vi "hmi_simRK4serial_variador_2port.vi"() -> ()   [LabVIEW 2017]
uses:
  Control 6.ctl
  <vilib>/Utility/miscctls.llb/LVBoundsTypeDef.ctl
  <vilib>/Instr/_visa.llb/VISA Configure Serial Port (Instr).vi
  <vilib>/MakerHub/LINX/LMH-LINX.lvlib
panel:
  in  "Iniciar fuga":bool
  out "ftselec2":dbl
  out "ftselec1":dbl
  out "Q2":dbl
  out "Q1":dbl
  in  "Simulacion":bool caption="Monitoreo"
  in  "Velocidad":i32(slide) scale=0.0..8333.0
  out "Tiempo":dbl caption="seg" format="%.1f"
  out "Periodo":dbl format="%#_3g"
  in  "FUGA 1":bool
  in  "FUGA 2":bool
  in  "Encendido":bool
  in  "stop":bool
  in  "GUARDAR DATOS EN EXCEL":bool
  in  "Puerto BOMBA":refnum<visa-resource-name>="COM3"
  in  "Puerto sensores":refnum<visa-resource-name>="COM3"
  out "time array":dbl[](array[numeric])
  in  "Tab Control":T1(tab)
  out "Presion de entrada":dbl caption="PSI"
  out "Boolean 2":bool
  out "Boolean":bool
  out "FT1":bool(c317)
  out "valvula 1":bool
  out "valvula 2":bool
  out "TEE 02":bool
  out "TUBERIA 1IN TRAMO 02":bool(c317)
  out "TEE1":bool
  out "Multi-Segment Pipe 2":T2
  out "Multi-Segment Pipe 3":bool(c317)
  out "Multi-Segment Pipe 4":bool(c317)
  out "FT2":bool(c317)
  out "FT 1":dbl caption="L/min"
  out "67.5°":bool
  out "FT 2":dbl caption="L/min"
  out "67.5° 3":bool
  out "45° 3":bool
  out "22.5° 3":bool
  out "90° 3":bool
  out "SENSOR FLUJO 3":bool
  out "45°":bool
  out "22.5°":bool
  out "90°":bool
  out "TANQUE\n FLUIDO:AGUA":dbl(slide) scale=0.0..100.0
  out "SENSOR FLUJO":bool
  out "BOMBA 1/2 HP":bool
  out "codo90":bool
  out "Presion de salida":dbl caption="PSI"
  out "Freq2":dbl
  out "Freq1":dbl
  out "Cluster":T3
  in  "Tab Control 3":enum32{"CAUDAL", "PRESION"}(tab)
  out "Flujo de entrada y salida":cluster{dbl[], dbl[]}[](graph) caption="TRANSMISORES DE FLUJO"
  out "Presion entrada y salida":cluster{dbl[], dbl[]}(graph) caption="TRANSMISORES DE PRESION (PSI)"
  out "Entrada":dbl
  out "Salida":dbl
  in  "Rango de grafica en X":i16(slide)=100 caption="seg" scale=0.0..200.0
  in  "Tab Control 2":T4(tab)
  out "SIMULACION DE Q1 y Q2":cluster{dbl[], dbl[]}[](graph)
  out "SIMULACION DE H2":cluster{"time array":dbl[], dbl[]}(graph)
  in  "Flujo de entrada":dbl=28.44 format="%#_13g"
  in  "Flujo de salida":dbl=26.1 format="%#_13g"
  in  "Rango de grafica":i16(slide)=100 scale=0.0..100.0
  # "INTERFAZ GRAFICA PARA EL MONITOREO DE UN TUBERÍA HIDRÁULICA"
  # "Configuración de comunicación"
  # "Control de Bomba"
  # "Alarmas de detección"
  # "PVC  1\" FLUJO: AGUA"
  # "PVC  1/2\" FLUJO: AGUA"
  # "FUGA 1"
  # "PVC  1/2\" FLUJO: AGUA"
  # "FUGA 2"
  # "PVC  1\" FLUJO: AGUA"
  # "2.5 m"
  # "6 m"
  # "Sensores de Flujo"
  # "Condiciones iniciales"
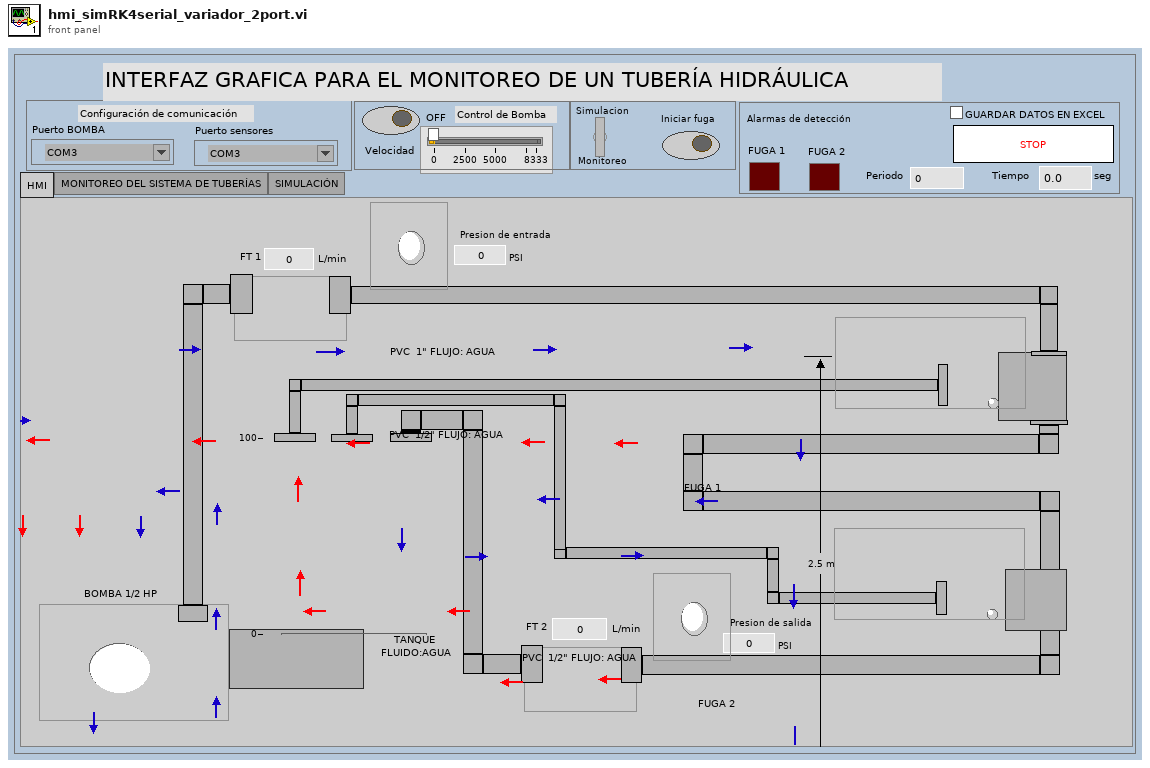
[diagram p1: front panel]
types:
  T1 = enum32{"HMI", "MONITOREO DEL SISTEMA DE TUBERÍAS", "SIMULACIÓN"}
  T2 = typedef "Control 6.ctl" = bool
  T3 = cluster{"FLUJO DE ENTRADA":dbl, "FLUJO DE SALIDA":dbl, "VOLUMEN 1 (L) ":dbl, "VOLUMEN 2 (L) ":dbl}
  T4 = enum32{"FLUJO DE ENTRADA Y SALIDA", "PRESION DE SALIDA"}
  T5 = typedef "LVBoundsTypeDef.ctl" = cluster{"Width":u32, "Height":u32}
  T6 = cluster{"index":i32, "index 2":i32, "index 3":i32, "index 4":i32, "index 5":i32, "index 6":i32, i32, i32}
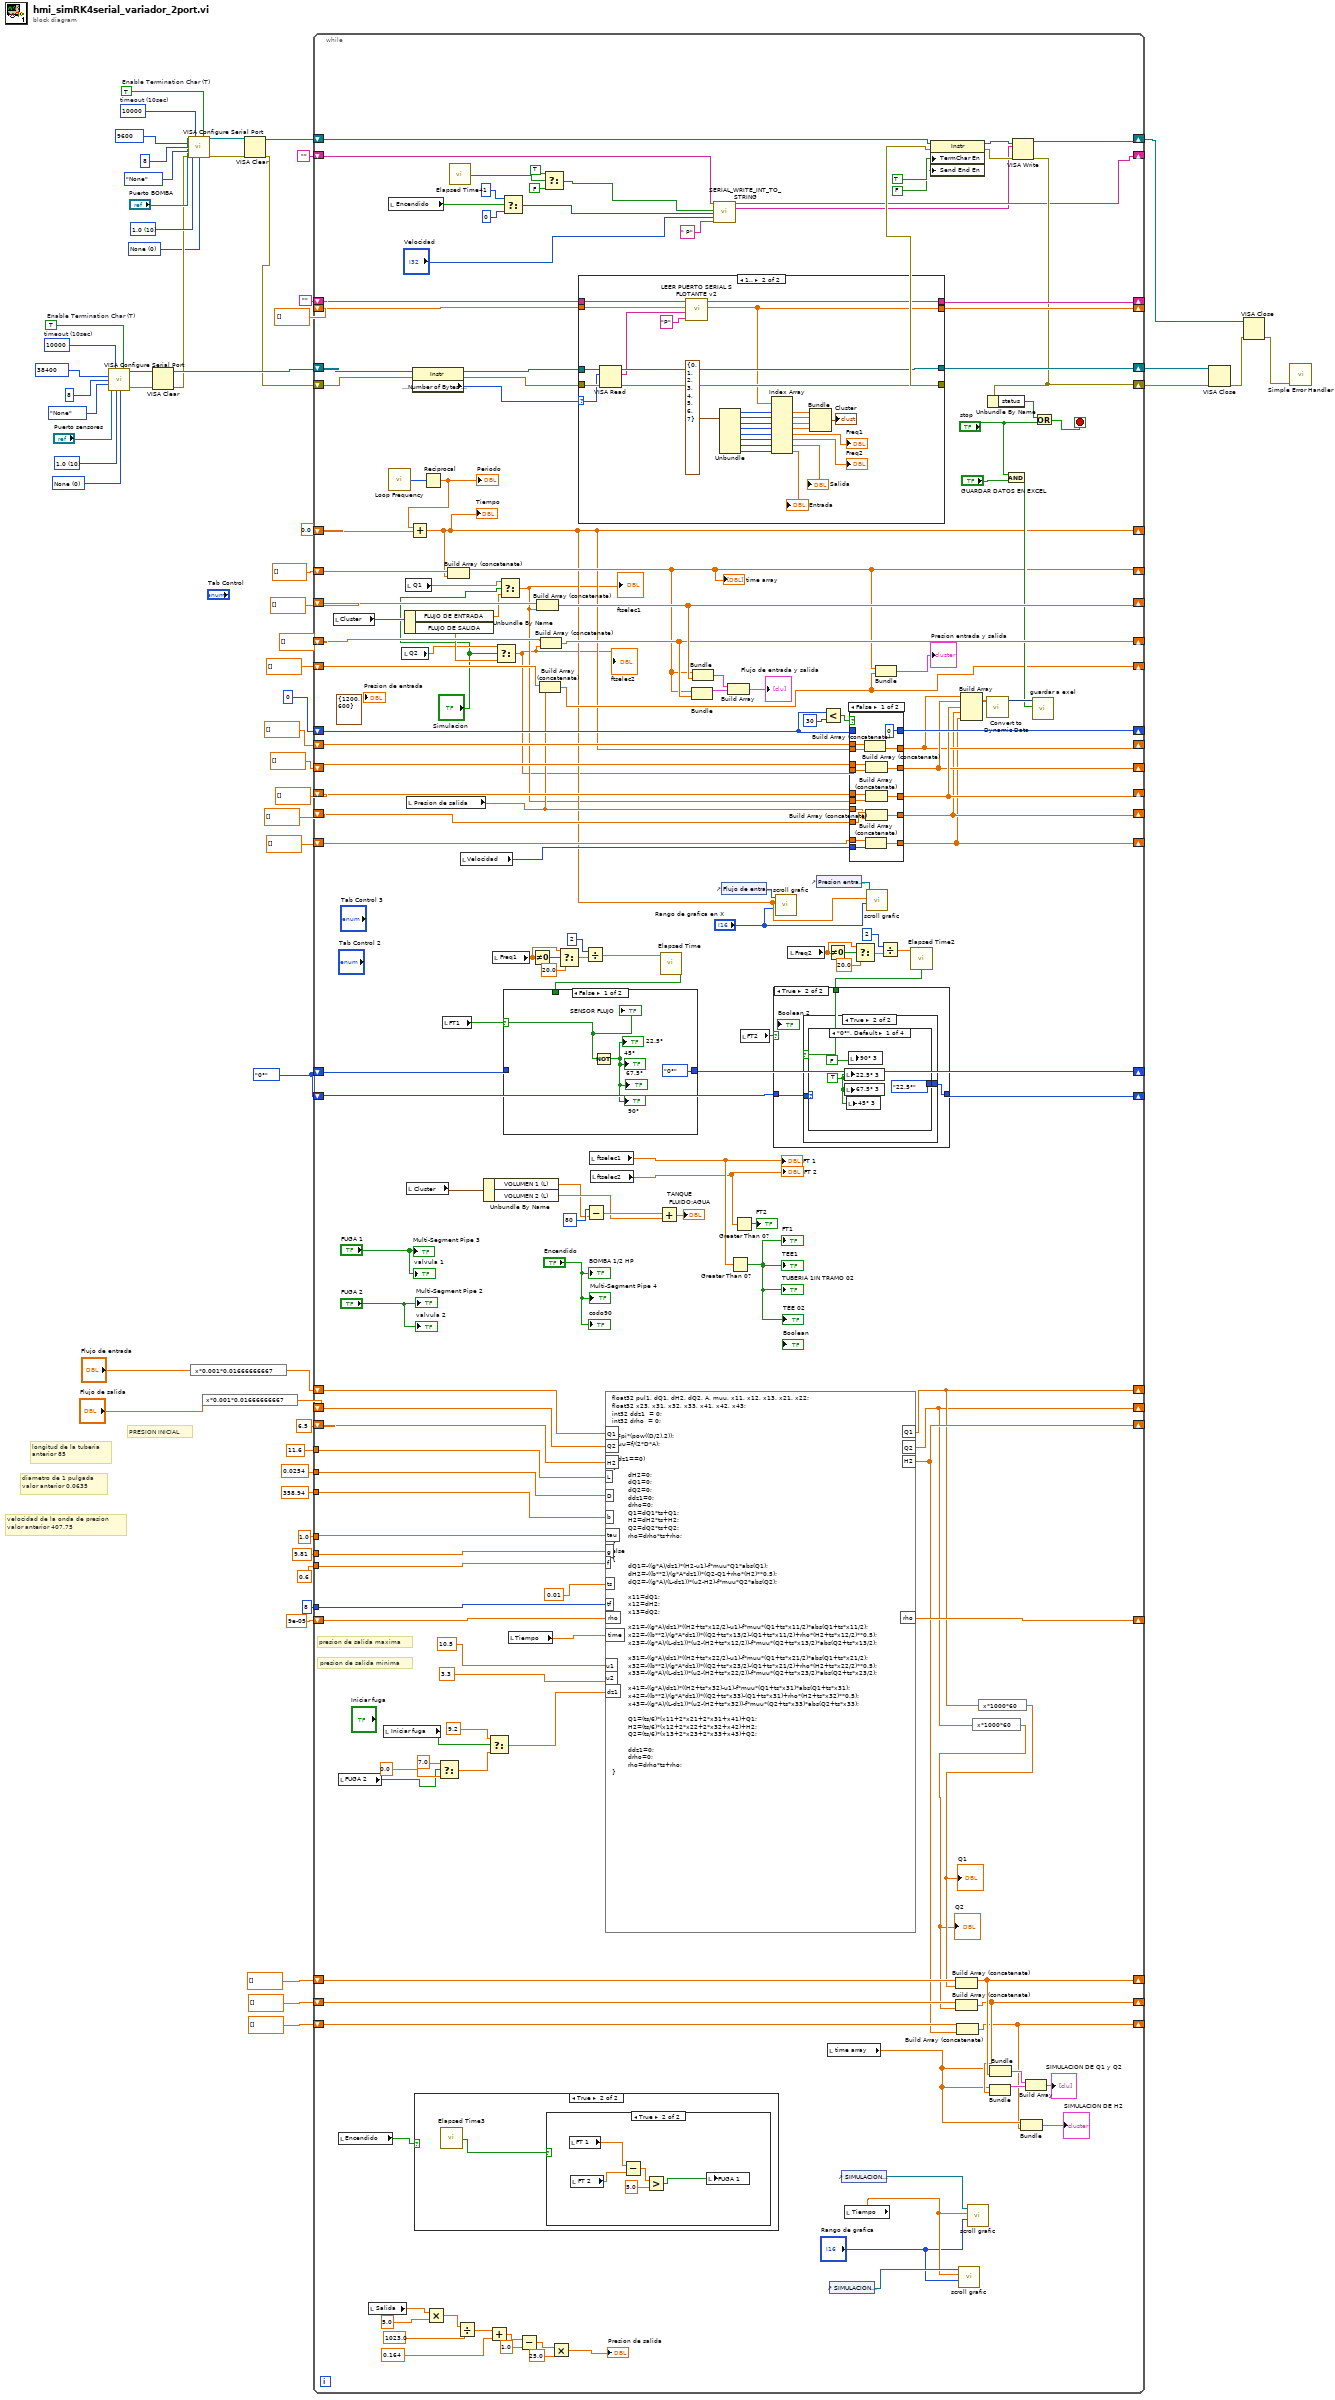
[diagram p0: block diagram]
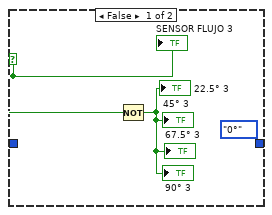
[diagram p4: hidden frame]
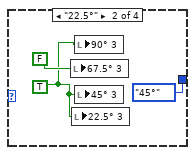
[diagram p6: hidden frame]
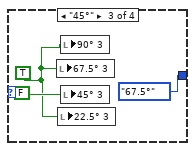
[diagram p7: hidden frame]
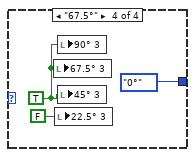
[diagram p8: hidden frame]
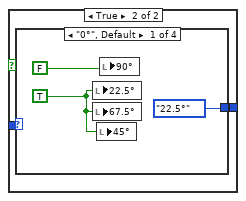
[diagram p10: hidden frame]
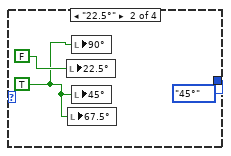
[diagram p11: hidden frame]
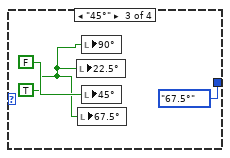
[diagram p12: hidden frame]
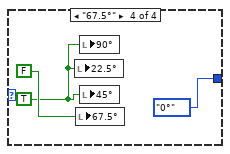
[diagram p13: hidden frame]
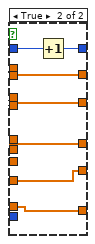
[diagram p14: hidden frame]
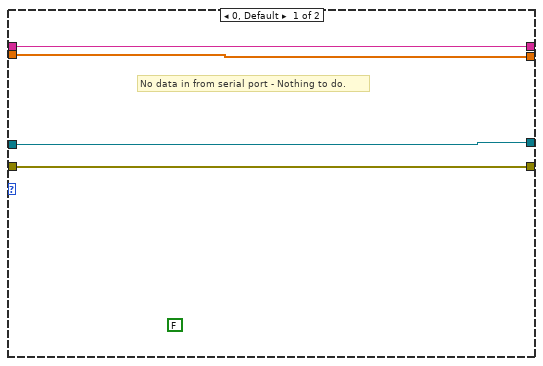
[diagram p15: hidden frame]
diagram:
  w18 = 9600 items=["9600"=9600, "19200"=19200, "38400"=38400, "57600"=57600, "74880"=74880, "115200"=115200] ("BaudRate")
  w21 = u16 10 items=["1.0"=10, "1.5"=15, "2.0"=20] ("stop bits (10: 1 bit)")
  w9 = u16 0 items=["None", "XON/XOFF", "RTS/CTS", "XON/XOFF & RTS/CTS", "DTR/DSR", "XON/XOFF & DTR/DSR"] ("flow control (0:none)")
  w23 = TRUE  # Enable Termination Char (T)
  w24 = u32 10000  # timeout (10sec)
  w40 = 38400 items=["9600"=9600, "19200"=19200, "38400"=38400, "57600"=57600, "74880"=74880, "115200"=115200] ("BaudRate")
  w39 = enum16{"0°", "22.5°", "45°", "67.5°"}."0°"
  w52 = u16 10 items=["1.0"=10, "1.5"=15, "2.0"=20] ("stop bits (10: 1 bit)")
  w53 = u16 0 items=["None", "XON/XOFF", "RTS/CTS", "XON/XOFF & RTS/CTS", "DTR/DSR", "XON/XOFF & DTR/DSR"] ("flow control (0:none)")
  w58 = TRUE  # Enable Termination Char (T)
  w59 = u32 10000  # timeout (10sec)
  (unwired) T5 {"Width"=1200, "Height"=600} ("Tab Control Pane Dimension")
  # "PRESION INICIAL"
  # "longitud de la tuberia\nanterior 85"
  # "velocidad de la onda de presion \nvalor anterior 407.75"
  # "diametro de 1 pulgada \nvalor anterior 0.0635"
  n1 = call-poly "VISA Configure Serial Port"("VISA resource name"="Puerto sensores", "timeout (10sec)"=w59, "Enable Termination\nChar (T)"=w58, "baud rate (9600)"=w40, "data bits (8)"=u16 8 ("Data bits (8)"), "parity (0:none)"=enum16{"None", "Odd", "Even", "Mark", "Space"}."None" ("Parity (0:none)"), "stop bits (10: 1 bit)"=w52, "flow control (0:none)"=w53) -> ("VISA resource name out"=w56:refnum<visa-resource-name>, "error out"=w57:errorcluster)  [unwired: 6 in]
  n2 = VISA Clear(VISA resource name=w56, error in (no error)=w57) -> (VISA resource name out=w55:refnum<visa-resource-name>, error out=w15:errorcluster)
  n3 = call-poly "VISA Configure Serial Port"("VISA resource name"="Puerto BOMBA", "timeout (10sec)"=w24, "Enable Termination\nChar (T)"=w23, "baud rate (9600)"=w18, "data bits (8)"=u16 8 ("Data bits (8)"), "parity (0:none)"=enum16{"None", "Odd", "Even", "Mark", "Space"}."None" ("Parity (0:none)"), "error in (no error)"=w15, "stop bits (10: 1 bit)"=w21, "flow control (0:none)"=w9) -> ("VISA resource name out"=w17:refnum<visa-resource-name>, "error out"=w14:errorcluster)  [unwired: 5 in]
  n4 = expression code="x*0.001*0.01666666667"("Flujo de entrada") -> (w3:dbl)
  n5 = expression code="x*0.001*0.01666666667"("Flujo de salida") -> (w2:dbl)
  n6 = VISA Clear(VISA resource name=w17, error in (no error)=w14) -> (VISA resource name out=w16:refnum<visa-resource-name>, error out=w13:errorcluster)
  n7 = while {
    shift-right: [w94] -> _
    shift-left: dbl[] [] -> [w223]
    shift-right: [w80] -> _
    shift-left: 0.0 -> [w224]
    shift-right: [w216] -> _
    shift-left: dbl[] [] -> [w221]
    shift-right: [w203] -> _
    shift-left: dbl[] [] -> [w222]
    shift-right: [w213] -> _
    shift-left: 0 -> [w214]
    shift-right: [w208] -> _
    shift-left: dbl[] [] -> [w211]
    shift-right: [w209] -> _
    shift-left: dbl[] [] -> [w210]
    shift-right: [w207] -> _
    shift-left: dbl[] [] -> [w212]
    shift-right: [w125] -> w60
    shift-left: w13 -> [w127]
    shift-right: [w147] -> w41
    shift-left: w55 -> [w227]
    shift-right: [w193] -> _
    shift-left: w39 -> [w192]
    shift-right: [w175] -> _
    shift-left: w39 -> [w184]
    shift-right: [w171] -> _
    shift-left: "" -> [w172]
    shift-right: [w169] -> _
    shift-left: dbl[] [] -> [w170]
    tunnel: 0.6 ("input variable") -> [w167]
    tunnel: 9.81 ("input variable") -> [w166]
    tunnel: 1.0 ("input variable") -> [w165]
    tunnel: 358.94 ("input variable") -> [w164]
    tunnel: 0.0254 ("D") -> [w163]
    tunnel: 11.6 ("L") -> [w162]
    shift-right: [w90] -> _
    shift-left: w3 -> [w161]
    shift-right: [w88] -> _
    shift-left: w2 -> [w160]
    shift-right: [w143] -> _
    shift-left: 6.5 -> [w159]
    shift-right: [w157] -> _
    shift-left: 9e-05 -> [w158]
    tunnel: 8 -> [w156]
    shift-right: [w139] -> _
    shift-left: dbl[] [] -> [w146]
    shift-right: [w138] -> _
    shift-left: dbl[] [] -> [w145]
    shift-right: [w134] -> _
    shift-left: dbl[] [] -> [w144]
    shift-right: [w128] -> w10
    shift-left: w16 -> [w129]
    shift-right: [w122] -> _
    shift-left: "" -> [w123]
    shift-right: [w96] -> _
    shift-left: dbl[] [] -> [w110]
    shift-right: [w95] -> _
    shift-left: dbl[] [] -> [w109]
    shift-right: [w91] -> _
    shift-left: dbl[] [] -> [w93]
    stop <- w168 stop-if-true
    # "presion de salida minima"
    # "presion de salida maxima"
    n8 = local read "Cluster"() -> (w202:T3)
    n9 = local read "FUGA 2"() -> (w149:bool)
    n10 = local read "Encendido"() -> (w113:bool)
    n11 = local read "Salida"() -> (w106:dbl)
    n12 = local read "Iniciar fuga"() -> (w150:bool)
    n13 = local read "Encendido"() -> (w117:bool)
    n14 = call <vilib>:"Loop Frequency.vi"() -> ("Loop Rate (Hz)"=w218:u32)
    n15 = local read "Q2"() -> (w64:dbl)
    n16 = Unbundle By Name(w202) -> ("FLUJO DE ENTRADA"=w69:dbl, "FLUJO DE SALIDA"=w67:dbl)
    n17 = local read "Q1"() -> (w65:dbl)
    n18 = local read "Presion de salida"() -> (w92:dbl)
    n19 = local read "Cluster"() -> (w195:T3)
    n20 = property class="Instr"(reference=w227, error in=w127) -> (reference out=w229:refnum<visa-resource-name>, error out=w228:errorcluster, "Serial Settings:Number of Bytes at Serial Port"=w226:u32)
    n21 = case shown="True" w113 {
      frame False {
      }
      frame True {
        n22 = call "Elapsed Time3"() -> ("Time has Elapsed"=w230:bool)  [unwired: 12 in, 7 out]
        n23 = case shown="True" w230 {
          frame False {
          }
          frame True {
            n24 = local read "FT 1"() -> (w235:dbl)
            n25 = local read "FT 2"() -> (w234:dbl)
            n26 = Subtract(x=w235, y=w234) -> (x-y=w233:dbl)
            n27 = Greater?(x=w233, y=5.0) -> (0:w231:bool)
            n28 = local write "FUGA 1"(w231) -> ()
          }
        }
      }
    }
    n29 = Reciprocal(x=w218) -> (1/x=w220:dbl)
    "Periodo" <- w220
    n30 = Add(x=w220, y=w224) -> (x+y=w80:dbl)
    "Tiempo" <- w80
    n31 = Multiply(x=w106, y=5.0) -> (x*y=w104:dbl)
    n32 = Select(t=7.0, s=w149, f=0.0) -> (s? t:f=w154:dbl)
    n33 = local read "FT1"() -> (w194:bool)
    n34 = Build Array (concatenate)(w223, w80) -> (w94:dbl[])
    "time array" <- w94
    n35 = call "Elapsed Time4"() -> ("Time has Elapsed"=w86:bool)  [unwired: 12 in, 7 out]
    n36 = Divide(x=w104, y=1023.0) -> (x/y=w103:dbl)
    n37 = local read "Velocidad"() -> (w108:i32)
    n38 = Unbundle By Name(w195) -> ("VOLUMEN 1 (L)"=w173:dbl, "VOLUMEN 2 (L)"=w196:dbl)
    n39 = Add(x=w103, y=0.164) -> (x+y=w101:dbl)
    n40 = Select(t=9.2, s=w150, f=w154) -> (s? t:f=w151:dbl)
    n41 = local read "Freq1"() -> (w190:dbl)
    n42 = Select(t=w64, s="Simulacion", f=w67) -> (s? t:f=w66:dbl)
    "ftselec2" <- w66
    n43 = Select(t=w65, s="Simulacion", f=w69) -> (s? t:f=w68:dbl)
    "ftselec1" <- w68
    n44 = Select(t=1, s=w117, f=0) -> (s? t:f=w114:i32)
    n45 = local read "Tiempo"() -> (w148:dbl)
    n46 = Subtract(x=w101, y=1.0) -> (x-y=w99:dbl)
    n47 = Not Equal To 0?(x=w190) -> (x != 0?=w191:bool)
    n48 = Build Array (concatenate)(w221, w68) -> (w216:dbl[])
    n49 = Build Array (concatenate)(w93, w92) -> (w91:dbl[])
    n50 = Build Array (concatenate)(w222, w66) -> (w203:dbl[])
    n51 = Select(t=TRUE, s=w86, f=FALSE) -> (s? t:f=w83:bool)
    n52 = Multiply(x=w99, y=25.0) -> (x*y=→"Presion de salida":dbl)
    n53 = Select(t=w190, s=w191, f=20.0) -> (s? t:f=w188:dbl)
    n54 = case shown="1.." w226 {
      selector: w226 -> [_ w329]
      tunnel: [w303 w333] -> w126
      tunnel: [w304 w332] -> w147
      tunnel: w229 -> [w304 w331]
      tunnel: w228 -> [w303 w330]
      tunnel: w172 -> [w302 w319]
      tunnel: [w302 w318] -> w171
      tunnel: w170 -> [w301 w317]
      tunnel: [w301 w316] -> w169
      frame 0, Default {
        (unwired) FALSE
        # "No data in from serial port - Nothing to do."
      }
      frame 1.. {
        n55 = VISA Read(VISA resource name=w331, byte count=w329, error in (no error)=w330) -> (VISA resource name out=w332:refnum<visa-resource-name>, read buffer=w320:string, error out=w333:errorcluster)  [unwired: 1 out]
        n56 = call <userlib>:"LEER PUERTO SERIAL S FLOTANTE v2.vi"("caracter terminador"="P" ("regular expression"), "read buffer"=w320, "buffer de datos"=w317, "buffer in"=w319) -> ("salida datos numericos"=w316:dbl[], "buffer out"=w318:string)  [unwired: 1 in, 1 out]
        n57 = Unbundle(T6 {"index"=0, "index 2"=1, "index 3"=2, "index 4"=3, "index 5"=4, "index 6"=5, 6, 7}) -> ("index"=w314:i32, "index 2"=w313:i32, "index 3"=w312:i32, "index 4"=w311:i32, "index 5"=w310:i32, "index 6"=w309:i32, w308:i32, w307:i32)
        n58 = Index Array(array=w316, index #1=w314, index #2=w313, index #3=w312, index #4=w311, index #5=w310, index #6=w309, index #7=w308, index #8=w307) -> (element #1=w327:dbl, element #2=w326:dbl, element #3=w324:dbl, element #4=w325:dbl, element #5=→"Freq1":dbl, element #6=→"Freq2":dbl, element #7=→"Salida":dbl, element #8=→"Entrada":dbl)
        n59 = Bundle(w327, w326, w324, w325) -> (→"Cluster":cluster{dbl, dbl, dbl, dbl})  [unwired: 1 in]
      }
    }
    n60 = Divide(x=i8 2, y=w188) -> (x/y=w187:dbl)
    n61 = Subtract(x=80, y=w173) -> (x-y=w197:dbl)
    n62 = local read "ftselec1"() -> (w62:dbl)
    "FT 1" <- w62
    n63 = local read "ftselec2"() -> (w61:dbl)
    "FT 2" <- w61
    n64 = formula code="float32 pul1, dQ1, dH2, dQ2, A, muu, x11, x12, x13, x21, x22;\nfloat32 x23, x31, x32, x33, x41, x42, x43;\nint32 ddz1  = 0;\nint32 drho  = 0;\n\nA=pi*(pow((D/2),2));\nmuu=f/(2*D*A);\n\nif(dz1==0)\n{\n        dH2=0;\n        dQ1=0;\n        dQ2=0;\n        ddz1=0;\n        drho=0;\n        Q1=dQ1*ts+Q1;\n        H2=dH2*ts+H2;    \n        Q2=dQ2*ts+Q2;\n        rho=drho*ts+rho;\n}\nelse \n{\n        dQ1=-((g*A)/dz1)*(H2-u1)-f*muu*Q1*abs(Q1);\n        dH2=-((b**2)/(g*A*dz1))*(Q2-Q1+rho*(H2)**0.5);\n        dQ2=-((g*A)/(L-dz1))*(u2-H2)-f*muu*Q2*abs(Q2);\n        \n        x11=dQ1;\n        x12=dH2;\n        x13=dQ2;\n        \n        x21=-((g*A)/dz1)*((H2+ts*x12/2)-u1)-f*muu*(Q1+ts*x11/2)*abs(Q1+ts*x11/2);\n        x22=-((b**2)/(g*A*dz1))*((Q2+ts*x13/2)-(Q1+ts*x11/2)+rho*(H2+ts*x12/2)**0.5);\n        x23=-((g*A)/(L-dz1))*(u2-(H2+ts*x12/2))-f*muu*(Q2+ts*x13/2)*abs(Q2+ts*x13/2);\n        \n        x31=-((g*A)/dz1)*((H2+ts*x22/2)-u1)-f*muu*(Q1+ts*x21/2)*abs(Q1+ts*x21/2);\n        x32=-((b**2)/(g*A*dz1))*((Q2+ts*x23/2)-(Q1+ts*x21/2)+rho*(H2+ts*x22/2)**0.5);\n        x33=-((g*A)/(L-dz1))*(u2-(H2+ts*x22/2))-f*muu*(Q2+ts*x23/2)*abs(Q2+ts*x23/2);\n        \n        x41=-((g*A)/dz1)*((H2+ts*x32)-u1)-f*muu*(Q1+ts*x31)*abs(Q1+ts*x31);\n        x42=-((b**2)/(g*A*dz1))*((Q2+ts*x33)-(Q1+ts*x31)+rho*(H2+ts*x32)**0.5);\n        x43=-((g*A)/(L-dz1))*(u2-(H2+ts*x32))-f*muu*(Q2+ts*x33)*abs(Q2+ts*x33);\n        \n        Q1=(ts/6)*(x11+2*x21+2*x31+x41)+Q1;\n        H2=(ts/6)*(x12+2*x22+2*x32+x42)+H2;\n        Q2=(ts/6)*(x13+2*x23+2*x33+x43)+Q2;\n        \n        ddz1=0;\n        drho=0;\n        rho=drho*ts+rho;\n}"("L"=w162, "D"=w163, "b"=w164, "tau"=w165, "g"=w166, "Q1"=w161, "Q2"=w160, "f"=w167, "ts"=0.01 ("input variable"), "tf"=w156, "rho"=w158, "H2"=w159, "time"=w148, "u1"=10.5, "u2"=3.3, "dz1"=w151) -> ("rho"=w157:dbl, "Q1"=w90:dbl, "Q2"=w88:dbl, "H2"=w143:dbl)
    n65 = Add(x=w197, y=w196) -> (x+y=→"TANQUE\n FLUIDO:AGUA":dbl)
    n66 = call "Elapsed Time"("Time Target (s)"=w187) -> ("Time has Elapsed"=w185:bool)  [unwired: 11 in, 7 out]
    n67 = case shown="False" w194 {
      selector: w194 -> [w259 _]
      tunnel: w192 -> [_ w262]
      tunnel: [enum16{"0°", "22.5°", "45°", "67.5°"}."0°" w261] -> w193
      tunnel: w185 -> [_ w260]
      frame False {
        n68 = Not(x=w259) -> (.not. x?=→"90°" →"22.5°" →"45°" →"67.5°":bool)
        "SENSOR FLUJO" <- w259
      }
      frame True {
        n69 = case shown="False" w260 {
          tunnel: w262 -> [w263 w265]
          tunnel: [w263 w264] -> w261
          frame False {
          }
          frame True {
            n70 = case shown="\"0°\", Default" w265 {
              tunnel: [enum16{"0°", "22.5°", "45°", "67.5°"}."22.5°" enum16{"0°", "22.5°", "45°", "67.5°"}."45°" enum16{"0°", "22.5°", "45°", "67.5°"}."67.5°" enum16{"0°", "22.5°", "45°", "67.5°"}."0°"] -> w264
              frame "0°", Default {
                w266 = TRUE
                n71 = local write "22.5°"(w266) -> ()
                n72 = local write "67.5°"(w266) -> ()
                n73 = local write "45°"(w266) -> ()
                n74 = local write "90°"(FALSE) -> ()
              }
              frame "22.5°" {
                w269 = TRUE
                n75 = local write "22.5°"(FALSE) -> ()
                n76 = local write "67.5°"(w269) -> ()
                n77 = local write "90°"(w269) -> ()
                n78 = local write "45°"(w269) -> ()
              }
              frame "45°" {
                w272 = TRUE
                n79 = local write "22.5°"(w272) -> ()
                n80 = local write "67.5°"(w272) -> ()
                n81 = local write "90°"(w272) -> ()
                n82 = local write "45°"(FALSE) -> ()
              }
              frame "67.5°" {
                w275 = TRUE
                n83 = local write "22.5°"(w275) -> ()
                n84 = local write "67.5°"(FALSE) -> ()
                n85 = local write "90°"(w275) -> ()
                n86 = local write "45°"(w275) -> ()
              }
            }
          }
        }
      }
    }
    n87 = Bundle(w94, w203) -> (w137:cluster{dbl[], dbl[]})  [unwired: 1 in]
    n88 = Bundle(w94, w216) -> (w219:cluster{dbl[], dbl[]})  [unwired: 1 in]
    n89 = call <userlib>:"SERIAL_WRITE_INT_TO_STRING.vi"("buffer in"=w123, "ENVIAR"=w83, "bomba on/off"=w114, "tiempo"="Velocidad", "fin de cadena"=" P") -> ("buffer out"=w122:string, "int to string out"=w121:string)  [unwired: 7 in, 2 out]
    n90 = control-ref of="Flujo de entrada y salida"() -> (w142:refnum<vi>)
    n91 = Build Array(w219, w137) -> (→"Flujo de entrada y salida":cluster{dbl[], dbl[]}[])
    n92 = Greater Than 0?(x=w62) -> (x > 0?=→"TUBERIA 1IN TRAMO 02" →"TEE1" →"TEE 02" →"FT1":bool)
    n93 = Greater Than 0?(x=w61) -> (x > 0?=→"FT2":bool)
    n94 = local read "FT2"() -> (w176:bool)
    n95 = call <userlib>:"scroll grafic.vi"("Rango de grafica"="Rango de grafica en X", "tiempo"=w80, "XYGraph in"=w142) -> ()  [unwired: 9 in]
    n96 = local read "Freq2"() -> (w182:dbl)
    n97 = control-ref of="Presion entrada y salida"() -> (w75:refnum<vi>)
    n98 = Less?(x=w214, y=u32 30) -> (x < y?=w204:bool)
    n99 = Not Equal To 0?(x=w182) -> (x != 0?=w183:bool)
    n100 = local read "time array"() -> (w135:dbl[])
    n101 = control-ref of="SIMULACION DE H2"() -> (w76:refnum<vi>)
    n102 = control-ref of="SIMULACION DE Q1 y Q2"() -> (w73:refnum<vi>)
    n103 = local read "Tiempo"() -> (w72:dbl)
    n104 = case shown="False" w204 {
      tunnel: w214 -> [_ w300]
      tunnel: [u32 0 w299] -> w213
      tunnel: w212 -> [w292 w296]
      tunnel: w66 -> [w290 _]
      tunnel: [w293 w298] -> w208
      tunnel: w211 -> [w291 w298]
      tunnel: w68 -> [w288 _]
      tunnel: w210 -> [w289 w297]
      tunnel: [w287 w297] -> w209
      tunnel: [w286 w296] -> w207
      tunnel: w80 -> [w285 _]
      tunnel: w110 -> [w283 w295]
      tunnel: [w282 w295] -> w96
      tunnel: w92 -> [w281 _]
      tunnel: w109 -> [w280 w294]
      tunnel: [w279 w294] -> w95
      tunnel: w108 -> [w278 _]
      frame False {
        n105 = Build Array (concatenate)(w292, w285) -> (w286:dbl[])
        n106 = Build Array (concatenate)(w280, w278) -> (w279:dbl[])
        n107 = Build Array (concatenate)(w291, w290) -> (w293:dbl[])
        n108 = Build Array (concatenate)(w289, w288) -> (w287:dbl[])
        n109 = Build Array (concatenate)(w283, w281) -> (w282:dbl[])
      }
      frame True {
        n110 = Increment(x=w300) -> (x+1=w299:u32)
      }
    }
    n111 = Select(t=w182, s=w183, f=20.0) -> (s? t:f=w180:dbl)
    n112 = call <userlib>:"scroll grafic.vi"("Rango de grafica"="Rango de grafica en X", "tiempo"=w80, "XYGraph in"=w75) -> ()  [unwired: 9 in]
    n113 = Bundle(w94, w91) -> (→"Presion entrada y salida":cluster{dbl[], dbl[]})  [unwired: 1 in]
    n114 = Divide(x=i8 2, y=w180) -> (x/y=w179:dbl)
    n115 = call "Elapsed Time2"("Time Target (s)"=w179) -> ("Time has Elapsed"=w177:bool)  [unwired: 11 in, 7 out]
    n116 = case shown="True" w176 {
      selector: w176 -> [w238 _]
      tunnel: w184 -> [_ w241]
      tunnel: [enum16{"0°", "22.5°", "45°", "67.5°"}."0°" w240] -> w175
      tunnel: w177 -> [_ w239]
      frame False {
        n117 = Not(x=w238) -> (.not. x?=→"90° 3" →"22.5° 3" →"45° 3" →"67.5° 3":bool)
        "SENSOR FLUJO 3" <- w238
      }
      frame True {
        n118 = case shown="True" w239 {
          tunnel: w241 -> [w242 w244]
          tunnel: [w242 w243] -> w240
          frame False {
          }
          frame True {
            n119 = case shown="\"0°\", Default" w244 {
              tunnel: [enum16{"0°", "22.5°", "45°", "67.5°"}."22.5°" enum16{"0°", "22.5°", "45°", "67.5°"}."45°" enum16{"0°", "22.5°", "45°", "67.5°"}."67.5°" enum16{"0°", "22.5°", "45°", "67.5°"}."0°"] -> w243
              frame "0°", Default {
                w245 = TRUE
                n120 = local write "22.5° 3"(w245) -> ()
                n121 = local write "67.5° 3"(w245) -> ()
                n122 = local write "45° 3"(w245) -> ()
                n123 = local write "90° 3"(FALSE) -> ()
              }
              frame "22.5°" {
                w248 = TRUE
                n124 = local write "67.5° 3"(FALSE) -> ()
                n125 = local write "22.5° 3"(w248) -> ()
                n126 = local write "90° 3"(w248) -> ()
                n127 = local write "45° 3"(w248) -> ()
              }
              frame "45°" {
                w251 = TRUE
                n128 = local write "67.5° 3"(w251) -> ()
                n129 = local write "22.5° 3"(w251) -> ()
                n130 = local write "90° 3"(w251) -> ()
                n131 = local write "45° 3"(FALSE) -> ()
              }
              frame "67.5°" {
                w254 = TRUE
                n132 = local write "67.5° 3"(w254) -> ()
                n133 = local write "22.5° 3"(FALSE) -> ()
                n134 = local write "90° 3"(w254) -> ()
                n135 = local write "45° 3"(w254) -> ()
              }
            }
          }
        }
      }
    }
    n136 = property class="Instr"(reference=w129, error in=w126, "TermChar En"=TRUE ("Message Based Settings:Termination Character Enable"), "Send End En"=FALSE ("Message Based Settings:Send End Enable")) -> (reference out=w131:refnum<visa-resource-name>, error out=w130:errorcluster)
    n137 = Build Array (concatenate)(w144, w143) -> (w134:dbl[])
    n138 = call <userlib>:"scroll grafic.vi"("Rango de grafica"="Rango de grafica", "tiempo"=w72, "XYGraph in"=w76) -> ()  [unwired: 9 in]
    n139 = Build Array(w207, w208, w209, w96, w95) -> (w205:dbl[][])
    n140 = call <userlib>:"scroll grafic.vi"("Rango de grafica"="Rango de grafica", "tiempo"=w72, "XYGraph in"=w73) -> ()  [unwired: 9 in]
    n141 = expression code="x*1000*60"(w88) -> (w87:dbl)
    "Q2" <- w87
    n142 = Build Array (concatenate)(w145, w87) -> (w138:dbl[])
    n143 = expression code="x*1000*60"(w90) -> (w89:dbl)
    "Q1" <- w89
    n144 = Build Array (concatenate)(w146, w89) -> (w139:dbl[])
    n145 = call "Convert to Dynamic Data"("2D Array"=w205) -> ("Dynamic Data Type"=w206:dynamicdata)  [unwired: 3 in]
    n146 = Bundle("time array"=w135, w138) -> (w140:cluster{"time array":dbl[], dbl[]})  [unwired: 1 in]
    n147 = Bundle("time array"=w135, w139) -> (w141:cluster{"time array":dbl[], dbl[]})  [unwired: 1 in]
    n148 = And(x="stop", y="GUARDAR DATOS EN EXCEL") -> (x .and. y?=w120:bool)
    n149 = VISA Write(VISA resource name=w131, write buffer=w121, error in (no error)=w130) -> (VISA resource name out=w128:refnum<visa-resource-name>, error out=w125:errorcluster)  [unwired: 1 out]
    n150 = Unbundle By Name(w125) -> ("status"=w225:bool)
    n151 = Bundle("time array"=w135, w134) -> (→"SIMULACION DE H2":cluster{"time array":dbl[], dbl[]})  [unwired: 1 in]
    n152 = Build Array(w141, w140) -> (→"SIMULACION DE Q1 y Q2":cluster{"time array":dbl[], dbl[]}[])
    n153 = call "guardar a exel"("Signals"=w206, "Enable"=w120) -> ()  [unwired: 15 in, 3 out]
    n154 = Or(x=w225, y="stop") -> (x .or. y?=w168:bool)
    "BOMBA 1/2 HP" <- "Encendido"
    "codo90" <- "Encendido"
    "Multi-Segment Pipe 4" <- "Encendido"
    "Multi-Segment Pipe 3" <- "FUGA 1"
    "valvula 2" <- "FUGA 2"
    "valvula 1" <- "FUGA 1"
    "Multi-Segment Pipe 2" <- "FUGA 2"
  }
  n155 = VISA Close(VISA resource name=w41, error in (no error)=w60) -> (error out=w12:errorcluster)
  n156 = VISA Close(VISA resource name=w10, error in (no error)=w12) -> (error out=w11:errorcluster)
  n157 = call <vilib>:"Simple Error Handler.vi"("error in (no error)"=w11) -> ()  [unwired: 4 in, 5 out]
